vi "meas_timing.vi"() -> (1 "meas cycle time":u32)   [LabVIEW 2012]
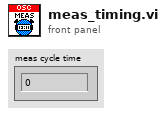
[diagram p1: front panel]
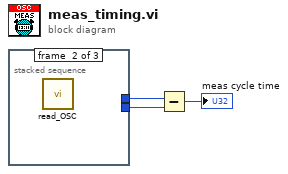
[diagram p0: block diagram]
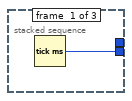
[diagram p2: hidden frame]
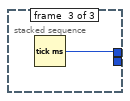
[diagram p3: hidden frame]
diagram:
  n1 = stacked-sequence {
    tunnel: [w4 _ _] -> w2
    tunnel: [_ _ w5] -> w3
    frame #0 {
      n2 = Tick Count (ms)() -> (millisecond timer value=w4:u32)
    }
    frame #1 {
      n3 = call "read_OSC.vi"() -> ()  [unwired: 5 in, 7 out]
    }
    frame #2 {
      n4 = Tick Count (ms)() -> (millisecond timer value=w5:u32)
    }
  }
  n5 = Subtract(x=w3, y=w2) -> (x-y=→"meas cycle time":u32)
